vi "ConfigureDigitalOutputs.vi"(0 "axis in":cluster{"keyHandle":u32, "nodeId":u16}={"keyHandle"=0, "nodeId"=1}, 7 "digital output configuration":T1={"digitalOutputNumber"=1, "configuration"=0, "state"=0, "mask"=0, "polarity"=0} {"polarity" items=["HighActive", "LowActive"]; "mask" items=["Disabled", "Enabled"]; "state" items=["Inactive", "Active"]; "configuration" items=["Ready"=0, "Position Compare"=1, "General Purpose A"=15, "General Purpose B"=14, "General Purpose C"=13, "General Purpose D"=12, "General Purpose E"=11, "General Purpose F"=10, "General Purpose G"=9, "General Purpose H"=8]}, 11 "error in (no error)":errorcluster) -> (4 "axis out":cluster{"keyHandle":u32, "nodeId":u16}={"keyHandle"=0, "nodeId"=1}, 15 "error out":errorcluster)   [LabVIEW 2017, in "maxonEPOS.lvlib"]
doc: "<B>ConfigureDigitalOutputs</B> writes the configuration parameters for a digital output to the device."
uses:
  Examples/maxonEPOS.lvlib
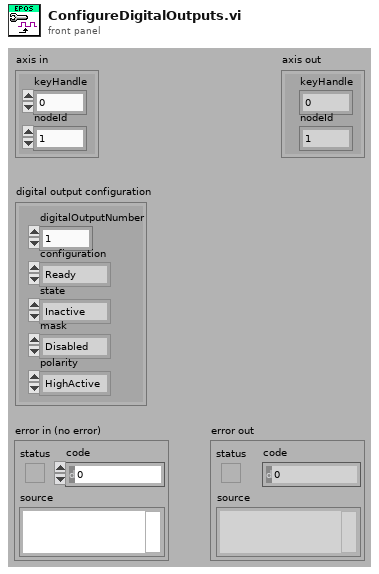
[diagram p1: front panel]
types:
  T1 = cluster{"digitalOutputNumber":u16, "configuration":u16, "state":i32, "mask":i32, "polarity":i32}
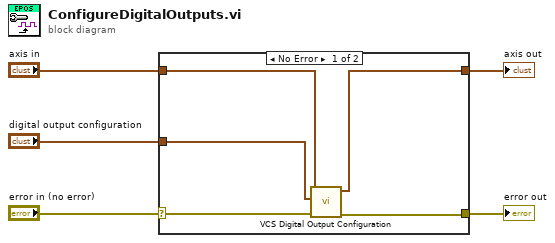
[diagram p0: block diagram]
diagram:
  n1 = case shown="No Error" "error in (no error)" {
    selector: "error in (no error)" -> [w9 w12]
    tunnel: [w8 w12] -> w4
    tunnel: [w7 w11] -> w3
    tunnel: "axis in" -> [w6 w11]
    tunnel: "digital output configuration" -> [w10 _]
    frame No Error {
      n2 = call "VCS Digital Output Configuration.vi"("error in (no error)"=w9, "output configuration"=w10, "axis in"=w6) -> ("error out"=w8:errorcluster, "axis out"=w7:cluster{"keyHandle":u32, "nodeId":u16})  [unwired: 7 in]
    }
    frame Error {
    }
  }
  "error out" <- w4
  "axis out" <- w3
